vi "Get autofocus component.vi"(8 "error in (no error)":errorcluster, 11 "Tomo in":refnum<class "Invivo_Tomo.lvclass">) -> (0 "error out":errorcluster, 2 "autofocus component":string, 3 "Tomo out":refnum<class "Invivo_Tomo.lvclass">)   [LabVIEW 2012, in "Invivo_Tomo.lvclass"]
uses:
  Invivo_Tomo.lvclass
  Invivo_Tomo.lvclass/Invivo_Tomo.ctl
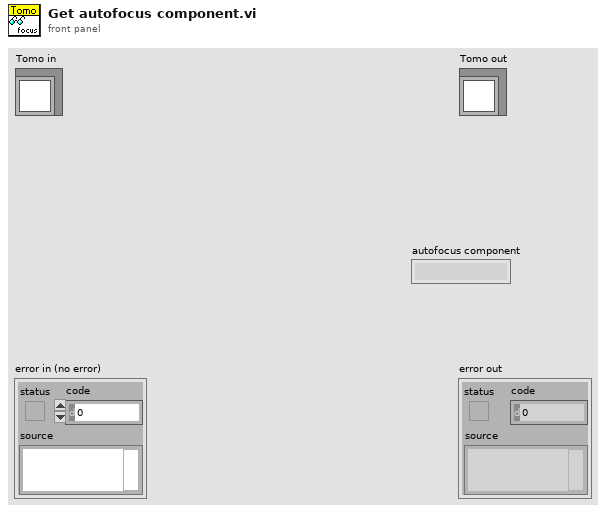
[diagram p1: front panel]
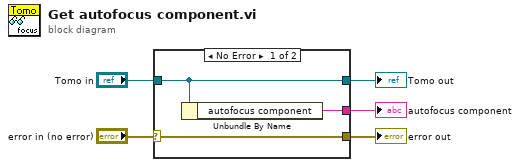
[diagram p0: block diagram]
diagram:
  n1 = case shown="No Error" "error in (no error)" {
    selector: "error in (no error)" -> [w8 w10]
    tunnel: [w8 w10] -> w4
    tunnel: [w7 w9] -> w2
    tunnel: "Tomo in" -> [w7 w9]
    tunnel: [w6 _] -> w1
    frame No Error {
      n2 = Unbundle By Name(w7) -> ("autofocus component"=w6:string)
    }
    frame Error {
    }
  }
  "error out" <- w4
  "Tomo out" <- w2
  "autofocus component" <- w1
